vi "D3DM_replot.vi"() -> ()   [LabVIEW 2013]
uses:
  <vilib>/Native 3D Graph/xcontrol/3DPC_SurfacePlot.xctl
  <userlib>/_OpenG.lib/array/array.llb/Remove Duplicates from 1D Array (DBL)__ogtk.vi
  <vilib>/Platform/NI_3dgraph.lvlib
panel:
  out "XYZ Array Size":i32[](array[numeric])
  out "text":string
  out "InRange":bool
  in  "3D Curve - Lorenz Attractor":refnum<k7>(container)
  in  "Simulation":bool
  in  "Least Dis":dbl=200.0
  in  "holder_length":dbl=87.37
  out "Title":string="      Distributed 3D Measurement Control Panel"
  in  "Log File Path":path=path "E:/Dropbox/StaredProject/Distributed3D/D3DM/raw_log.txt"
  in  "ArcStepThreshold":dbl=8000.0
  out "3D Graph":refnum<class "Base Datatype.lvclass">[](xcontrol)
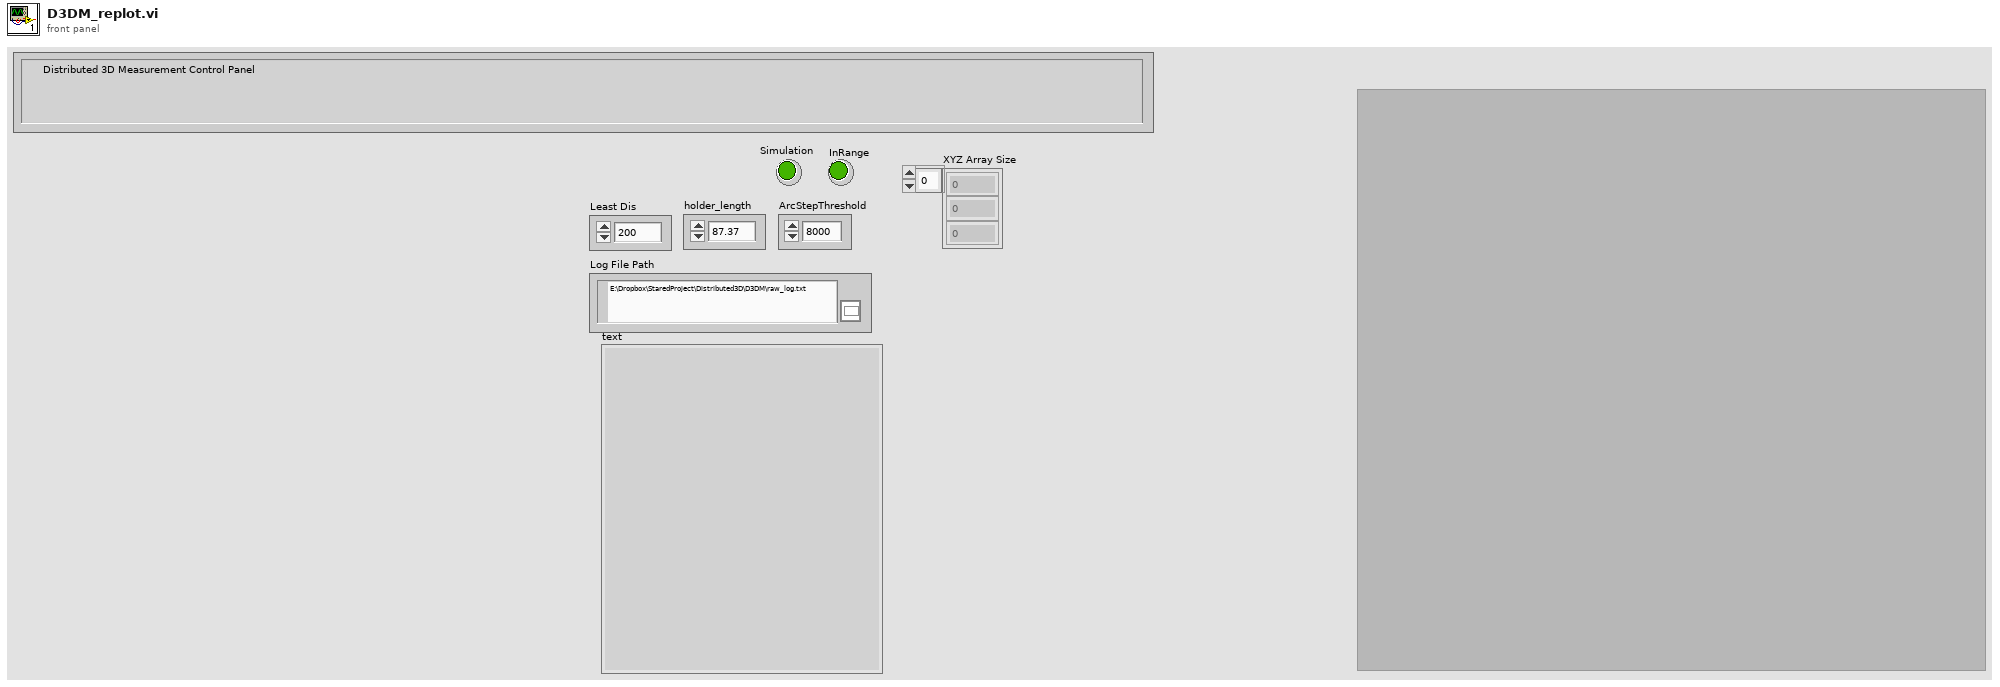
[diagram p1: front panel]
types:
  T1 = enum16{"open", "replace", "create", "open or create", "replace or create", "replace or create with confirmation"}
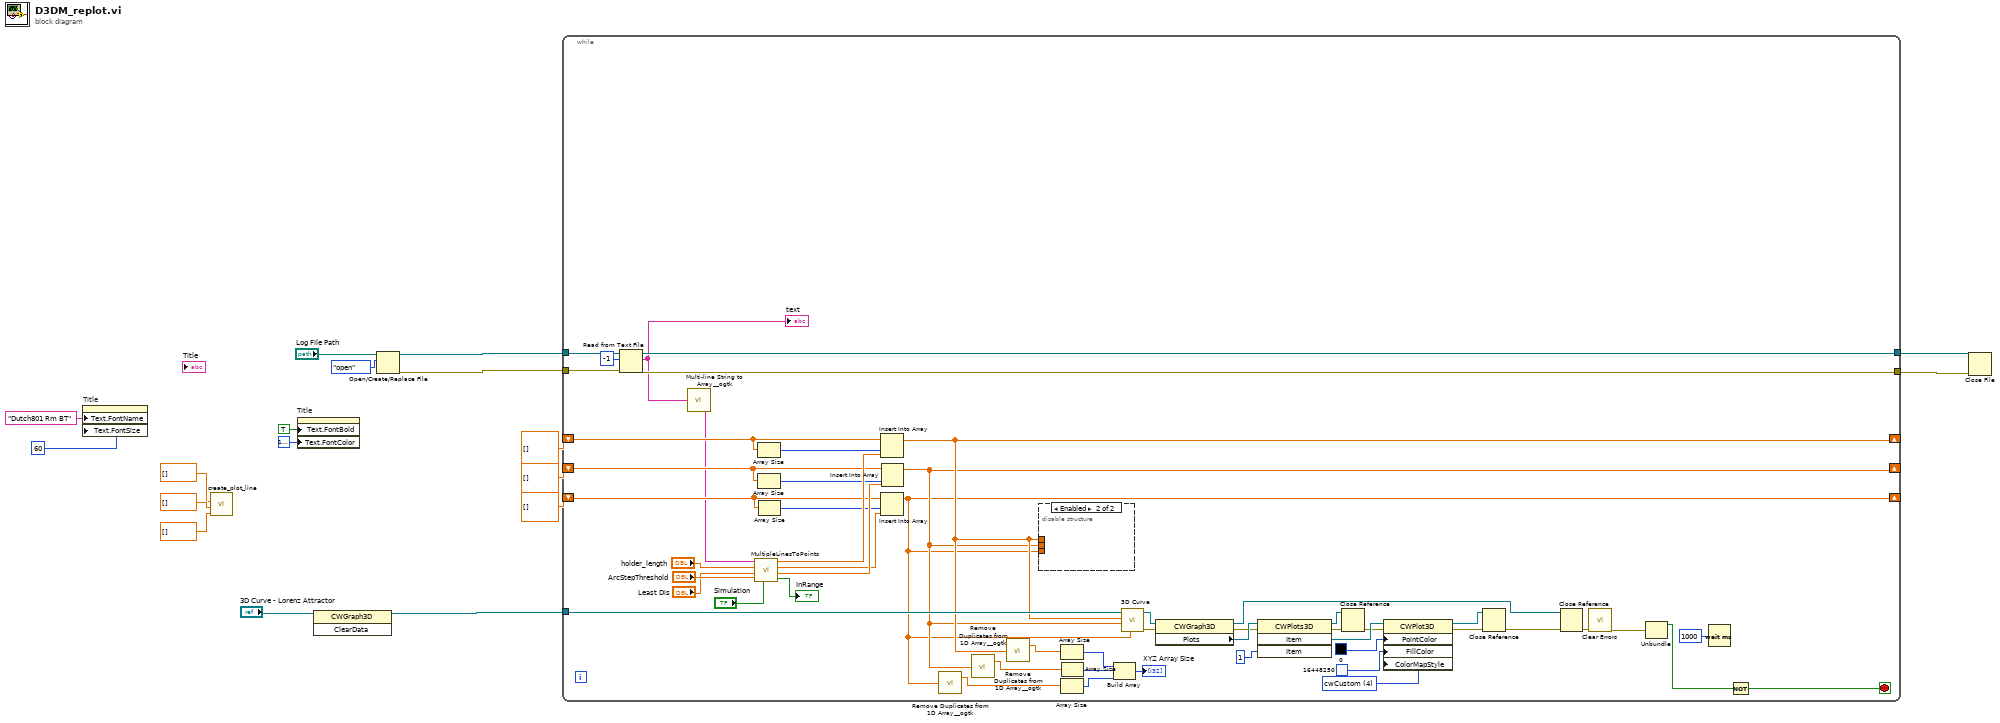
[diagram p0: block diagram]
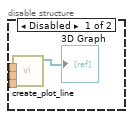
[diagram p2: hidden frame]
diagram:
  n1 = property on="Title" class="Str"("Text.FontName"="Dutch801 Rm BT" ("Text.Font:Name"), "Text.FontSize"=u32 60 ("Text.Font:Size")) -> ()  [unwired: 2 in, 2 out]
  n2 = call <vilib>:"create_plot_line.vi"("z vector"=dbl[] [], "y vector"=dbl[] [], "x vector"=dbl[] []) -> ()  [unwired: 8 in, 1 out]
  n3 = property on="Title" class="Str"("Text.FontBold"=TRUE ("Text.Font:Bold"), "Text.FontColor"=u32 16777222) -> ()  [unwired: 2 in, 2 out]
  n4 = invoke class="CWGraph3D" method="ClearData"(reference="3D Curve - Lorenz Attractor") -> (reference out=w6:refnum<k7>)  [unwired: 2 in, 2 out]
  n5 = Open/Create/Replace File(file path (use dialog)="Log File Path", operation (0:open)=T1."open") -> (refnum out=w16:refnum<file>, error out=w15:errorcluster)  [unwired: 4 in, 1 out]
  n6 = while {
    tunnel: w16 -> [w39]
    tunnel: w15 -> [w38]
    shift-right: [w24] -> _
    shift-left: dbl[] [] -> [w68]
    shift-right: [w23] -> _
    shift-left: dbl[] [] -> [w64]
    shift-right: [w22] -> _
    shift-left: dbl[] [] -> [w63]
    tunnel: w6 -> [w41]
    tunnel: [w36] -> w5
    tunnel: [w35] -> w4
    stop <- w25 stop-if-true
    w45 = 4 items=["cwNone", "cwShaded", "cwColorSpectrum", "cwGrayScale", "cwCustom"] ("ColorMapStyle")
    n7 = Read from Text File(file (use dialog)=w39, count=-1, error in=w38) -> (refnum out=w36:refnum<file>, text=w34:string, error out=w35:errorcluster)  [unwired: 1 in, 1 out]
    "text" <- w34
    n8 = call <userlib>:"Multi-line String to Array__ogtk.vi"("string"=w34) -> ("lines"=w33:string[])
    n9 = call "MultipleLinesToPoints.vi"("Sim"="Simulation", "Arc Threshold"="ArcStepThreshold", "Least Dis"="Least Dis", "holder_length"="holder_length", "lines"=w33) -> ("InRange"=→"InRange":bool, "y"=w70:dbl[], "z"=w69:dbl[], "x"=w71:dbl[])  [unwired: 1 in]
    n10 = Array Size(array=w68) -> (size(s)=w67:i32)
    n11 = Array Size(array=w64) -> (size(s)=w66:i32)
    n12 = Array Size(array=w63) -> (size(s)=w65:i32)
    n13 = Insert Into Array(array=w68, index=w67, new element=w71) -> (w24:dbl[])
    n14 = Insert Into Array(array=w63, index=w65, new element=w69) -> (w22:dbl[])
    n15 = Insert Into Array(array=w64, index=w66, new element=w70) -> (w23:dbl[])
    n16 = call-poly <userlib>:"Remove Duplicates from 1D Array__ogtk.vi"("Input Array"=w22) -> ("Output Array"=w21:dbl[])  [unwired: 1 out]
    n17 = call-poly <userlib>:"Remove Duplicates from 1D Array__ogtk.vi"("Input Array"=w23) -> ("Output Array"=w20:dbl[])  [unwired: 1 out]
    n18 = call-poly <userlib>:"Remove Duplicates from 1D Array__ogtk.vi"("Input Array"=w24) -> ("Output Array"=w19:dbl[])  [unwired: 1 out]
    n19 = disable-structure shown="Enabled" {
      disable-tunnel: w24 -> [w74 _]
      disable-tunnel: w23 -> [w73 _]
      disable-tunnel: w22 -> [w72 _]
      frame Disabled {
        n20 = call <vilib>:"create_plot_line.vi"("z vector"=w72, "y vector"=w73, "x vector"=w74) -> ("plots out"=→"3D Graph":refnum<class "Base Datatype.lvclass">[])  [unwired: 8 in]
      }
      frame Enabled {
      }
    }
    n21 = Array Size(array=w19) -> (size(s)=w31:i32)
    n22 = Array Size(array=w21) -> (size(s)=w29:i32)
    n23 = Array Size(array=w20) -> (size(s)=w30:i32)
    n24 = Build Array(w31, w30, w29) -> (→"XYZ Array Size":i32[])
    n25 = call <vilib>:"3D Curve.vi"("z vector"=w22, "y vector"=w23, "x vector"=w24, "3D graph"=w41) -> ("error out"=w59:errorcluster, "3D graph out"=w58:refnum<k7>)  [unwired: 6 in]
    n26 = property class="CWGraph3D"(reference=w58, error in=w59) -> (reference out=w49:refnum<k7>, error out=w57:errorcluster, "Plots"=w61:refnum<k7>)
    n27 = invoke class="CWPlots3D" method="Item"(reference=w61, error in=w57, "Item"=1) -> (reference out=w55:refnum<k7>, error out=w56:errorcluster, "Item"=w60:refnum<k7>)  [unwired: 1 in, 1 out]
    n28 = Close Reference(reference=w55, error in (no error)=w56) -> (error out=w54:errorcluster)
    n29 = property class="CWPlot3D"(reference=w60, error in=w54, "PointColor"=u32 0, "FillColor"=u32 16448250, "ColorMapStyle"=w45) -> (reference out=w52:refnum<k7>, error out=w53:errorcluster)
    n30 = Close Reference(reference=w52, error in (no error)=w53) -> (error out=w50:errorcluster)
    n31 = Close Reference(reference=w49, error in (no error)=w50) -> (error out=w51:errorcluster)
    n32 = call <vilib>:"Clear Errors.vi"("error in (no error)"=w51) -> ("error out"=w27:errorcluster)  [unwired: 6 in]
    n33 = Unbundle(w27) -> ("status"=w26:bool)  [unwired: 2 out]
    n34 = Wait (ms)(milliseconds to wait=u32 1000) -> ()  [unwired: 1 out]
    n35 = Not(x=w26) -> (.not. x?=w25:bool)
  }
  n36 = Close File(refnum=w5, error in=w4) -> ()  [unwired: 2 out]
